vi "Actor Core.vi"(8 "error in":errorcluster, 11 "TwoPaneViewManager In":refnum<class "TwoPaneViewManager.lvclass">) -> (0 "error out":errorcluster, 3 "Actor out":refnum<class "Actor.lvclass">)   [LabVIEW 2017, in "MVAExamples.lvlib" / "TwoPaneViewManager.lvclass"]
doc: "(<B>Filename</B>: Actor Framework.lvlib:Actor.lvclass:Actor Core.vi)\n\nReceives messages to the actor, reacts to them, and initiates any error handling that may shut the actor down.\n\nDescendant classes may override this VI to append parallel tasks for the actor to complete while it handles messages. Overrides use the Call Parent Method node.\n\n<License>\nCopyright © 2017 Composed Systems, LLC | All rights reserved\nwww.composed.io\n\nAuthor: Ethan Stern <ethan.stern@composed.io>\n\nThis software is provided \"AS IS\" WITHOUT WARRANTIES, either express or implied, AND IS FOR EDUCATIONAL PURPOSES ONLY.\n</License>"
uses:
  TwoPaneViewManager.lvclass
  gpm_packages/@cs/mva-viewable/Source/IViewable/ProtectedSubpanel/ProtectedSubpanel.lvclass
  gpm_packages/@cs/mva-viewable/Source/IViewManager/IViewManager/IViewManager.lvclass
  <vilib>/ActorFramework/Actor/Actor.lvclass
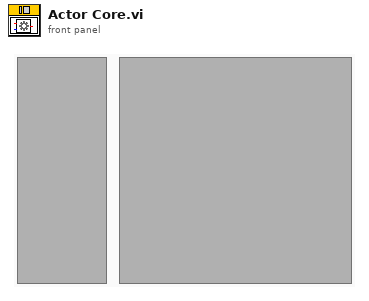
[diagram p1: front panel]
types:
  T1 = typedef "IViewable.lvlib/ProtectedSubpanel.lvclass/Protected Subpanel Reference.ctl" = refnum<data-value>
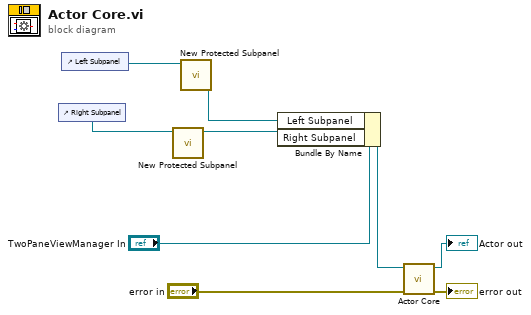
[diagram p0: block diagram]
diagram:
  n1 = control-ref of="Right Subpanel"() -> (w4:refnum<vi>)
  n2 = control-ref of="Left Subpanel"() -> (w5:refnum<vi>)
  n3 = call "New Protected Subpanel.vi"("SubPnl Refnum"=w4) -> ("Protected Subpanel"=w1:T1)  [unwired: 9 in, 1 out]
  n4 = call "New Protected Subpanel.vi"("SubPnl Refnum"=w5) -> ("Protected Subpanel"=w2:T1)  [unwired: 9 in, 1 out]
  n5 = Bundle By Name(cluster="TwoPaneViewManager In", "Left Subpanel"=w2, "Right Subpanel"=w1) -> (w3:refnum<class "TwoPaneViewManager.lvclass">)
  n6 = call-parent "Actor Core.vi"("error in"="error in", "IViewable In"=w3) -> ("error out"=→"error out":errorcluster, "Actor out"=→"Actor out":refnum<class "Actor.lvclass">)  [unwired: 8 in]
